vi "gfitsio-write-image-subset-u8-1d.vi"(6 "fpixel":i32[](array[numeric]), 8 "error in (no error)":errorcluster, 9 "data":u8[](array[numeric]), 11 "gfits refnum":T1) -> (0 "error out":errorcluster, 3 "dup gfits refnum":T1)   [LabVIEW 2014, in "gfitsio.lvlib"]
doc: "Write to a subset of the FITS data array. <B>fpixel</B> specifies the first pixel in the subset and must have the same number of elements as the image has dimensions. The data array will be written along the fastest changing dimensions of the image. This starts with NAXIS1 in the FITS file (column-major order) and in LabVIEW this starts with the last element in <b>fpixel</b> (row-major order)."
uses:
  gfitsio.lvlib
  gfitsio-refnum.ctl
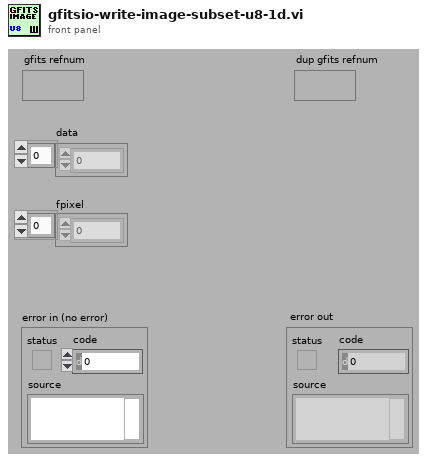
[diagram p1: front panel]
types:
  T1 = typedef "gfitsio.lvlib/gfitsio-refnum.ctl" = refnum<k1>
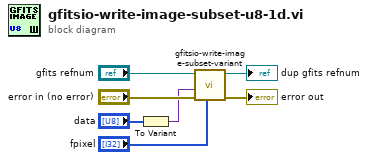
[diagram p0: block diagram]
diagram:
  n1 = To Variant(anything="data") -> (Variant=w1:variant)
  n2 = call "gfitsio-write-image-subset-variant.vi"("fpixel"="fpixel", "error in (no error)"="error in (no error)", "data"=w1, "gfits refnum"="gfits refnum") -> ("error out"=→"error out":errorcluster, "dup gfits refnum"=→"dup gfits refnum":T1)  [unwired: 6 in]
